vi "Nth Order EMA.vi"(0 "input":fxp<+/-,48,1>, 1 "reset":bool, 5 "order":i32, 7 "n_cutoff":i8, 9 "input valid":bool) -> (4 "output":fxp<+/-,48,1>, 10 "output valid":bool)   [LabVIEW 2018, in "NI PLL IP FPGA.lvlib"]
uses:
  NI PLL IP FPGA.lvlib
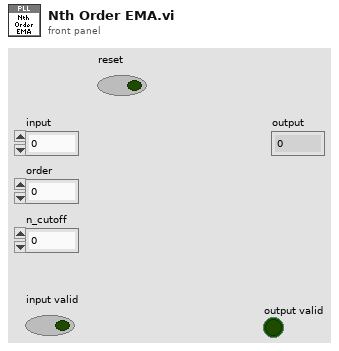
[diagram p1: front panel]
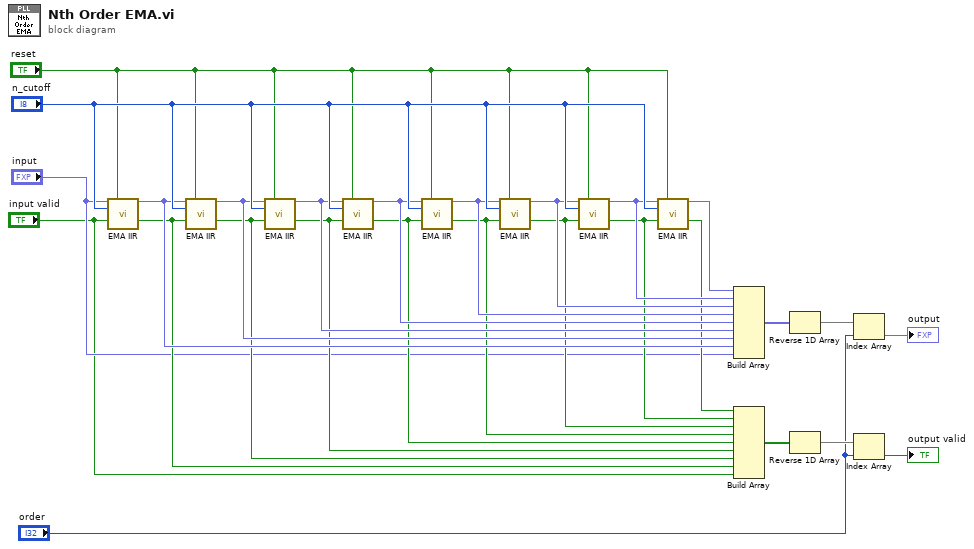
[diagram p0: block diagram]
diagram:
  n1 = call "EMA IIR.vi"("input"="input", "reset"="reset", "b_n"="n_cutoff", "input valid"="input valid") -> ("output"=w19:fxp<+/-,48,1>, "output valid"=w12:bool)  [unwired: 10 in]
  n2 = call "EMA IIR.vi"("input"=w19, "reset"="reset", "b_n"="n_cutoff", "input valid"=w12) -> ("output"=w20:fxp<+/-,48,1>, "output valid"=w13:bool)  [unwired: 10 in]
  n3 = call "EMA IIR.vi"("input"=w20, "reset"="reset", "b_n"="n_cutoff", "input valid"=w13) -> ("output"=w21:fxp<+/-,48,1>, "output valid"=w14:bool)  [unwired: 10 in]
  n4 = call "EMA IIR.vi"("input"=w21, "reset"="reset", "b_n"="n_cutoff", "input valid"=w14) -> ("output"=w22:fxp<+/-,48,1>, "output valid"=w15:bool)  [unwired: 10 in]
  n5 = call "EMA IIR.vi"("input"=w22, "reset"="reset", "b_n"="n_cutoff", "input valid"=w15) -> ("output"=w23:fxp<+/-,48,1>, "output valid"=w16:bool)  [unwired: 10 in]
  n6 = call "EMA IIR.vi"("input"=w23, "reset"="reset", "b_n"="n_cutoff", "input valid"=w16) -> ("output"=w24:fxp<+/-,48,1>, "output valid"=w17:bool)  [unwired: 10 in]
  n7 = call "EMA IIR.vi"("input"=w24, "reset"="reset", "b_n"="n_cutoff", "input valid"=w17) -> ("output"=w25:fxp<+/-,48,1>, "output valid"=w18:bool)  [unwired: 10 in]
  n8 = call "EMA IIR.vi"("input"=w25, "reset"="reset", "b_n"="n_cutoff", "input valid"=w18) -> ("output"=w26:fxp<+/-,48,1>, "output valid"=w11:bool)  [unwired: 10 in]
  n9 = Build Array(w26, w25, w24, w23, w22, w21, w20, w19, "input") -> (w10:fxp<+/-,48,1>[])
  n10 = Build Array(w11, w18, w17, w16, w15, w14, w13, w12, "input valid") -> (w9:bool[])
  n11 = Reverse 1D Array(array=w10) -> (reversed array=w8:fxp<+/-,48,1>[])
  n12 = Reverse 1D Array(array=w9) -> (reversed array=w7:bool[])
  n13 = Index Array(array=w8, index="order") -> (element=→"output":fxp<+/-,48,1>)
  n14 = Index Array(array=w7, index="order") -> (element=→"output valid":bool)
